vi "PWM_v2.vi"(8 "error in":errorcluster, 9 "Cycles":i32=10, 10 "duty cycle (%)":dbl=25.0 format="%0.2f", 11 "PWM Sel.":enum16{"1", "2", "3", "4", "5", "6"}(ring)) -> (0 "error out":errorcluster={"status"=FALSE, "code"=200040, "source"="Property Node (arg 1) in PWM_v1.vi"}, 3 "TS Result":dbl[](array[numeric]))   [LabVIEW 2022 SP3]
uses:
  <vilib>/DAQmx/write.llb/DAQmx Write (Analog 1D Wfm NChan NSamp).vi
  <vilib>/DAQmx/read.llb/DAQmx Read (Analog 1D Wfm NChan NSamp).vi
  <vilib>/DAQmx/create/channels.llb/DAQmx Create Channel (AO-Voltage-Basic).vi
  <vilib>/DAQmx/create/channels.llb/DAQmx Create Channel (AI-Voltage-Basic).vi
  <vilib>/DAQmx/configure/timing.llb/DAQmx Timing (Sample Clock).vi
  <vilib>/measure/mascope.llb/Amplitude and Levels N chan.vi
  <vilib>/DAQmx/miscellaneous.llb/DAQmx Fill In Error Info.vi
  <vilib>/measure/mascope.llb/Pulse Measurements N chan.vi
  <resource>/objmgr/daqmx.rc
  <vilib>/measure/NI_MAPro.lvlib
  <vilib>/measure/NI_MABase.lvlib
panel:
  out "period":dbl[](array[numeric]) format="%.2p"
  out "pulse duration":dbl[](array[numeric]) format="%.2p"
  out "duty cycle":dbl[](array[numeric]) format="%.2p"
  out "Amp Gain":dbl[](array[numeric])=[2.051898140791966]
  in  "Sample Rate":dbl=50000.0
  in  "Sample Clock Source AI":tag="OnboardClock"
  in  "Sample Mode AI":i32(ring)=10178 items=["Finite Samples"=10178, "Continuous Samples"=10123, "Hardware Timed Single Point"=12522]
  out "Amplitude Out":dbl[](array[numeric])=[4.854499013364962] format="%.2p"
  out "High Out":dbl[](array[numeric])=[4.863375920862381] format="%.2p"
  out "Low Out":dbl[](array[numeric])=[0.008876907497418828] format="%.2p"
  out "Amplitude In":dbl[](array[numeric])=[9.9609375] format="%.2p"
  out "Low In":dbl[](array[numeric])=[0.01953125] format="%.2p"
  out "High In":dbl[](array[numeric])=[9.98046875] format="%.2p"
  in  "Sample Mode AO":i32(ring)=10123 items=["Finite Samples"=10178, "Continuous Samples"=10123, "Hardware Timed Single Point"=12522]
  out "Output Waveform":waveform(dbl)[](graph)=[{"t0"=timestamp(3719340435.858088 s since 1904-01-01), "dt"=1.9999999999999998e-05, "Y"=array[500 elements], "attributes"=variant("NI_ChannelName"=variant(string "BONTS_Mod1/ai24"), "NI_UnitDescription"=variant(string "Volts"))}]
  out "Input Waveform":waveform(dbl)[](graph)=[{"t0"=timestamp(0 s since 1904-01-01), "dt"=2e-05, "Y"=[10.0, 10.0, 10.0, 10.0, 10.0, 10.0, 10.0, 10.0, 0.0, 0.0, 0.0, 0.0, 0.0, 0.0, 0.0, 10.0, 10.0, 10.0, 10.0, 10.0, 10.0, 10.0, 0.0, 0.0, 0.0, 0.0, 0.0, 0.0, 0.0, 10.0, 10.0, 10.0, 10.0, 10.0, 10.0, 10.0, 0.0, 0.0, 0.0, 0.0, 0.0, 0.0, 0.0, 10.0, 10.0, 10.0, 10.0, 10.0, 10.0, 10.0, 0.0, 0.0, 0.0, 0.0, 0.0, 0.0, 0.0, 0.0, 10.0, 10.0, 10.0, 10.0, 10.0, 10.0, 10.0, 0.0, 0.0, 0.0, 0.0, 0.0, 0.0, 0.0, 10.0, 10.0, 10.0, 10.0, 10.0, 10.0, 10.0, 0.0, 0.0, 0.0, 0.0, 0.0, 0.0, 0.0, 10.0, 10.0, 10.0, 10.0, 10.0, 10.0, 10.0, 0.0, 0.0, 0.0, 0.0, 0.0, 0.0, 0.0, 10.0, 10.0, 10.0, 10.0, 10.0, 10.0, 10.0, 10.0, 0.0, 0.0, 0.0, 0.0, 0.0, 0.0, 0.0, 10.0, 10.0, 10.0, 10.0, 10.0, 10.0, 10.0, 0.0, 0.0, 0.0, 0.0, 0.0, 0.0, 0.0, 10.0, 10.0, 10.0, 10.0, 10.0, 10.0, 10.0, 0.0, 0.0, 0.0, 0.0, 0.0, 0.0, 0.0, 10.0, 10.0, 10.0, 10.0, 10.0, 10.0, 10.0, 0.0, 0.0, 0.0, 0.0, 0.0, 0.0, 0.0, 0.0, 10.0, 10.0, 10.0, 10.0, 10.0, 10.0, 10.0, 0.0, 0.0, 0.0, 0.0, 0.0, 0.0, 0.0, 10.0, 10.0, 10.0, 10.0, 10.0, 10.0, 10.0, 0.0, 0.0, 0.0, 0.0, 0.0, 0.0, 0.0, 10.0, 10.0, 10.0, 10.0, 10.0, 10.0, 10.0, 0.0, 0.0, 0.0, 0.0, 0.0, 0.0, 0.0, 10.0, 10.0, 10.0, 10.0, 10.0, 10.0, 10.0, 10.0, 0.0, 0.0, 0.0, 0.0, 0.0, 0.0, 0.0, 10.0, 10.0, 10.0, 10.0, 10.0, 10.0, 10.0, 0.0, 0.0, 0.0, 0.0, 0.0, 0.0, 0.0, 10.0, 10.0, 10.0, 10.0, 10.0, 10.0, 10.0, 0.0, 0.0, 0.0, 0.0, 0.0, 0.0, 0.0, 10.0, 10.0, 10.0, 10.0, 10.0, 10.0, 10.0, 0.0, 0.0, 0.0, 0.0, 0.0, 0.0, 0.0, 0.0, 10.0, 10.0, 10.0, 10.0, 10.0, 10.0, 10.0, 0.0, 0.0, 0.0, 0.0, 0.0, 0.0, 0.0, 10.0, 10.0, 10.0, 10.0, 10.0, 10.0, 10.0, 0.0, 0.0, 0.0, 0.0, 0.0, 0.0, 0.0, 10.0, 10.0, 10.0, 10.0, 10.0, 10.0, 10.0, 0.0, 0.0, 0.0, 0.0, 0.0, 0.0, 0.0, 10.0, 10.0, 10.0, 10.0, 10.0, 10.0, 10.0, 10.0, 0.0, 0.0, 0.0, 0.0, 0.0, 0.0, 0.0, 10.0, 10.0, 10.0, 10.0, 10.0, 10.0, 10.0, 0.0, 0.0, 0.0, 0.0, 0.0, 0.0, 0.0, 10.0, 10.0, 10.0, 10.0, 10.0, 10.0, 10.0, 0.0, 0.0, 0.0, 0.0, 0.0, 0.0, 0.0, 10.0, 10.0, 10.0, 10.0, 10.0, 10.0, 10.0, 0.0, 0.0, 0.0, 0.0, 0.0, 0.0, 0.0, 0.0, 10.0, 10.0, 10.0, 10.0, 10.0, 10.0, 10.0, 0.0, 0.0, 0.0, 0.0, 0.0, 0.0, 0.0, 10.0, 10.0, 10.0, 10.0, 10.0, 10.0, 10.0, 0.0, 0.0, 0.0, 0.0, 0.0, 0.0, 0.0, 10.0, 10.0, 10.0, 10.0, 10.0, 10.0, 10.0, 0.0, 0.0, 0.0, 0.0, 0.0, 0.0, 0.0, 10.0, 10.0, 10.0, 10.0, 10.0, 10.0, 10.0, 10.0, 0.0, 0.0, 0.0, 0.0, 0.0, 0.0, 0.0, 10.0, 10.0, 10.0, 10.0, 10.0, 10.0, 10.0, 0.0, 0.0, 0.0, 0.0, 0.0, 0.0, 0.0, 10.0, 10.0, 10.0, 10.0, 10.0, 10.0, 10.0, 0.0, 0.0, 0.0, 0.0, 0.0, 0.0, 0.0, 10.0, 10.0, 10.0, 10.0, 10.0, 10.0, 10.0, 0.0, 0.0, 0.0, 0.0, 0.0, 0.0, 0.0, 0.0, 10.0, 10.0, 10.0, 10.0, 10.0, 10.0, 10.0, 0.0, 0.0, 0.0, 0.0, 0.0, 0.0, 0.0, 10.0, 10.0, 10.0, 10.0, 10.0, 10.0, 10.0, 0.0, 0.0, 0.0, 0.0, 0.0, 0.0, 0.0, 10.0, 10.0, 10.0, 10.0, 10.0, 10.0, 10.0, 0.0, 0.0, 0.0, 0.0, 0.0, 0.0, 0.0]}]
  in  "Sample Clock Source AO":tag="OnboardClock"
  out "Actual Sample Rate":dbl=50000.0 format="%0.2f"
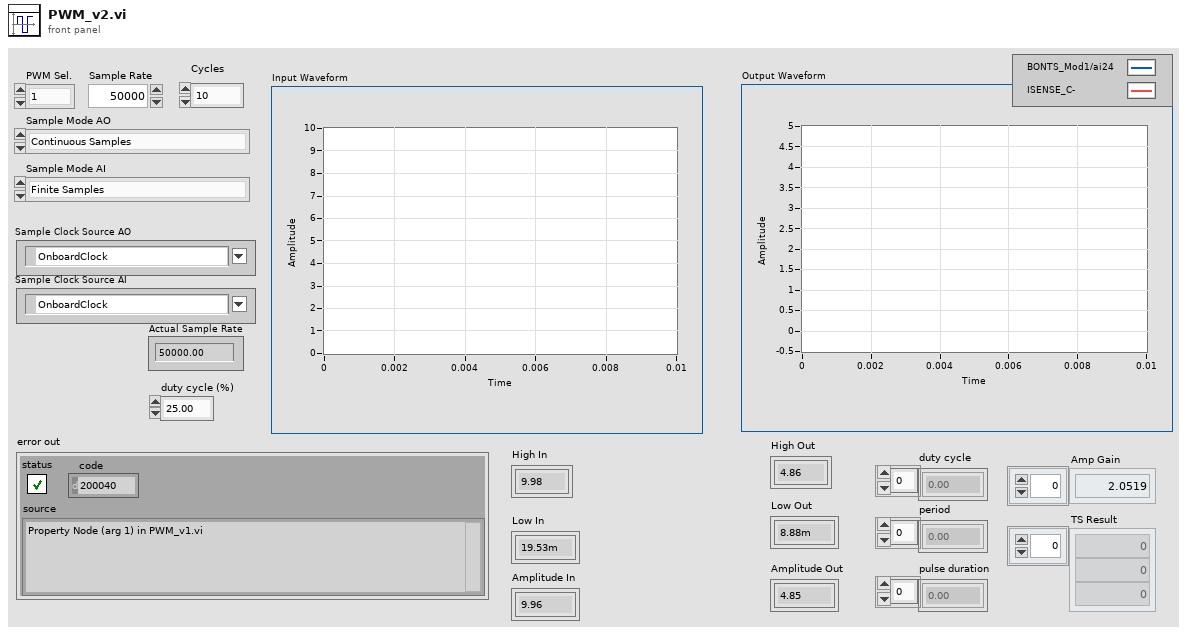
[diagram p1: front panel]
types:
  T1 = cluster{"Waveform Type":u16, "Amplitude":dbl, "Frequency":dbl}[]
  T2 = cluster{"Waveform Type":u16, "Amplitude":dbl, "Frequency":dbl}
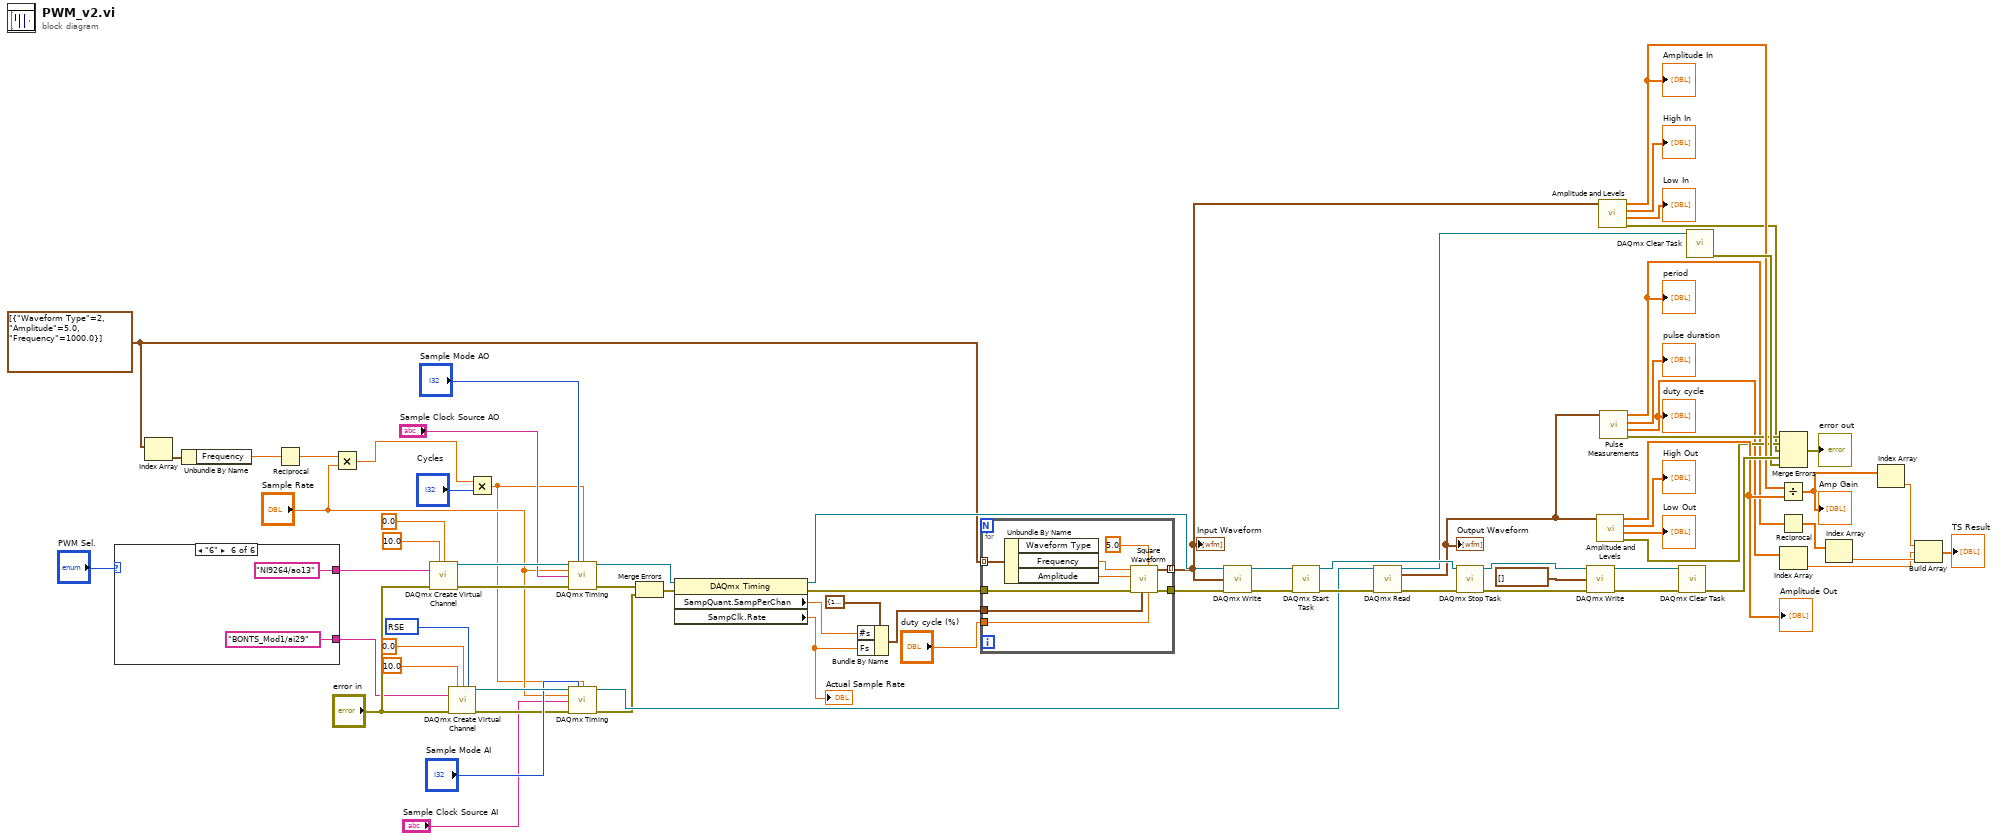
[diagram p0: block diagram]
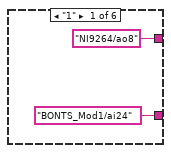
[diagram p2: hidden frame]
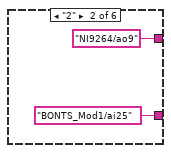
[diagram p3: hidden frame]
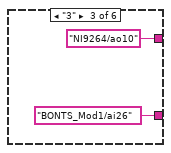
[diagram p4: hidden frame]
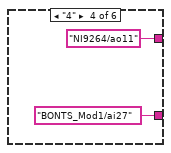
[diagram p5: hidden frame]
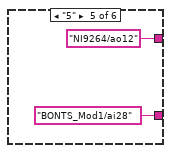
[diagram p6: hidden frame]
diagram:
  w22 = 10083 items=["Default"=-1, "RSE"=10083, "NRSE"=10078, "Differential"=10106, "Pseudodifferential"=12529] ("input terminal configuration")
  w8 = T1 [{"Waveform Type"=2, "Amplitude"=5.0, "Frequency"=1000.0}] ("Output Array")
  n1 = case shown="\"6\"" "PWM Sel." {
    tunnel: ["BONTS_Mod1/ai24" ("Read Channel") "BONTS_Mod1/ai25" ("Read Channel") "BONTS_Mod1/ai26" ("Read Channel") "BONTS_Mod1/ai27" ("Read Channel") "BONTS_Mod1/ai28" ("Read Channel") "BONTS_Mod1/ai29" ("Read Channel")] -> w31
    tunnel: ["NI9264/ao8" ("Write Channel") "NI9264/ao9" ("Write Channel") "NI9264/ao10" ("Write Channel") "NI9264/ao11" ("Write Channel") "NI9264/ao12" ("Write Channel") "NI9264/ao13" ("Write Channel")] -> w50
    frame "1" {
    }
    frame "2" {
    }
    frame "3" {
    }
    frame "4" {
    }
    frame "5" {
    }
    frame "6" {
    }
  }
  n2 = Index Array(array=w8) -> (element=w7:T2)  [unwired: 1 in]
  n3 = Unbundle By Name(w7) -> ("Frequency"=w6:dbl)
  n4 = Reciprocal(x=w6) -> (1/x=w5:dbl)
  n5 = Multiply(x=w5, y="Sample Rate") -> (x*y=w3:dbl)
  n6 = call-poly <vilib>:"DAQmx Create Virtual Channel.vi"("maximum value"=10.0, "minimum value"=0.0, "physical channels"=w50, "error in"="error in") -> ("task out"=w70:refnum<k21>, "error out"=w71:errorcluster)  [unwired: 10 in]
  n7 = call-poly <vilib>:"DAQmx Create Virtual Channel.vi"("maximum value"=10.0, "minimum value"=0.0, "input terminal configuration"=w22, "physical channels"=w31, "error in"="error in") -> ("task out"=w39:refnum<k21>, "error out"=w36:errorcluster)  [unwired: 9 in]
  n8 = Multiply(x=w3, y="Cycles") -> (x*y=w1:dbl)
  n9 = call-poly <vilib>:"DAQmx Timing.vi"("task/channels in"=w70, "sample mode"="Sample Mode AO", "samples per channel"=w1, "rate"="Sample Rate", "source"="Sample Clock Source AO", "error in"=w71) -> ("task out"=w51:refnum<k21>, "error out"=w34:errorcluster)  [unwired: 8 in]
  n10 = call-poly <vilib>:"DAQmx Timing.vi"("task/channels in"=w39, "sample mode"="Sample Mode AI", "samples per channel"=w1, "rate"="Sample Rate", "source"="Sample Clock Source AI", "error in"=w36) -> ("task out"=w40:refnum<k21>, "error out"=w33:errorcluster)  [unwired: 8 in]
  n11 = Merge Errors(w34, w33) -> (w35:errorcluster)
  n12 = property class="DAQmx Timing"(reference=w51, error in=w35) -> (reference out=w49:refnum<k21>, error out=w60:errorcluster, "SampQuant.SampPerChan"=w63:dbl, "SampClk.Rate"=w62:dbl)
  "Actual Sample Rate" <- w62
  n13 = Bundle By Name(cluster=cluster{"Fs":dbl, "#s":dbl} {"Fs"=1000.0, "#s"=1000.0} ("sampling info"), "#s"=w63, "Fs"=w62) -> (w67:cluster{"Fs":dbl, "#s":dbl})
  n14 = for {
    tunnel: w60 -> [w93]
    tunnel: w67 -> [w92]
    tunnel: [w91] -> w64
    tunnel: w8 -> [w90] mode=indexing
    tunnel: [w87] -> w26 mode=indexing
    tunnel: "duty cycle (%)" -> [w85]
    n15 = Unbundle By Name(w90) -> ("Frequency"=w89:dbl, "Amplitude"=w88:dbl)  [unwired: 1 out]
    n16 = call <vilib>:"Square Waveform.vi"("duty cycle (%)"=w85, "offset"=5.0, "sampling info"=w92, "error in (no error)"=w93, "amplitude"=w88, "frequency"=w89) -> ("error out"=w91:errorcluster, "signal out"=w87:waveform(dbl))  [unwired: 4 in]
  }
  "Input Waveform" <- w26
  n17 = call-poly <vilib>:"DAQmx Write.vi"("task/channels in"=w49, "data"=w26, "error in"=w64) -> ("task out"=w66:refnum<k21>, "error out"=w65:errorcluster)  [unwired: 10 in, 1 out]
  n18 = call <vilib>:"DAQmx Start Task.vi"("task/channels in"=w66, "error in"=w65) -> ("task out"=w61:refnum<k21>, "error out"=w59:errorcluster)  [unwired: 12 in]
  n19 = call-poly <vilib>:"DAQmx Read.vi"("task/channels in"=w40, "error in"=w59) -> ("task out"=w27:refnum<k21>, "data"=w21:waveform(dbl)[], "error out"=w58:errorcluster)  [unwired: 11 in]
  "Output Waveform" <- w21
  n20 = call <vilib>:"DAQmx Stop Task.vi"("task/channels in"=w61, "error in"=w58) -> ("task out"=w46:refnum<k21>, "error out"=w48:errorcluster)  [unwired: 12 in]
  n21 = call-poly <vilib>:"DAQmx Write.vi"("task/channels in"=w46, "data"=waveform(dbl)[] [], "error in"=w48) -> ("task out"=w45:refnum<k21>, "error out"=w47:errorcluster)  [unwired: 10 in, 1 out]
  n22 = call-poly <vilib>:"Amplitude and Levels.vi"("signal(s) in"=w21) -> ("error out"=w18:errorcluster, "low state level"=→"Low Out":dbl[], "high state level"=→"High Out":dbl[], "amplitude"=w24:dbl[])  [unwired: 7 in]
  "Amplitude Out" <- w24
  n23 = call-poly <vilib>:"Amplitude and Levels.vi"("signal(s) in"=w26) -> ("error out"=w17:errorcluster, "low state level"=→"Low In":dbl[], "high state level"=→"High In":dbl[], "amplitude"=w25:dbl[])  [unwired: 7 in]
  "Amplitude In" <- w25
  n24 = call-poly <vilib>:"Pulse Measurements.vi"("signal(s) in"=w21) -> ("error out"=w19:errorcluster, "duty cycle"=w15:dbl[], "pulse duration"=→"pulse duration":dbl[], "period"=w14:dbl[])  [unwired: 6 in, 1 out]
  "duty cycle" <- w15
  "period" <- w14
  n25 = call <vilib>:"DAQmx Clear Task.vi"("task in"=w45, "error in"=w47) -> ("error out"=w29:errorcluster)  [unwired: 13 in]
  n26 = call <vilib>:"DAQmx Clear Task.vi"("task in"=w27) -> ("error out"=w28:errorcluster)  [unwired: 14 in]
  n27 = Divide(x=w25, y=w24) -> (x/y=w16:dbl[])
  "Amp Gain" <- w16
  n28 = Reciprocal(x=w14) -> (1/x=w13:dbl[])
  n29 = Merge Errors(w19, w18, w17, w29, w28) -> (→"error out":errorcluster)
  n30 = Index Array(array=w15) -> (element=w11:dbl)  [unwired: 1 in]
  n31 = Index Array(array=w13) -> (element=w12:dbl)  [unwired: 1 in]
  n32 = Index Array(array=w16) -> (element=w10:dbl)  [unwired: 1 in]
  n33 = Build Array(w10, w11, w12) -> (→"TS Result":dbl[])
